vi "File Rename.vi"(10 "name or relative path":string="a.txt", 11 "path":path=path "C:/Users/tilin/Desktop/新文字文件.txt") -> ()   [LabVIEW 2019]
panel:
  out "appended path":path
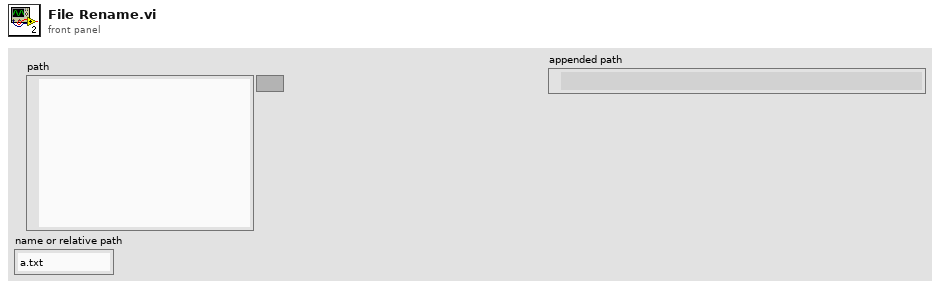
[diagram p1: front panel]
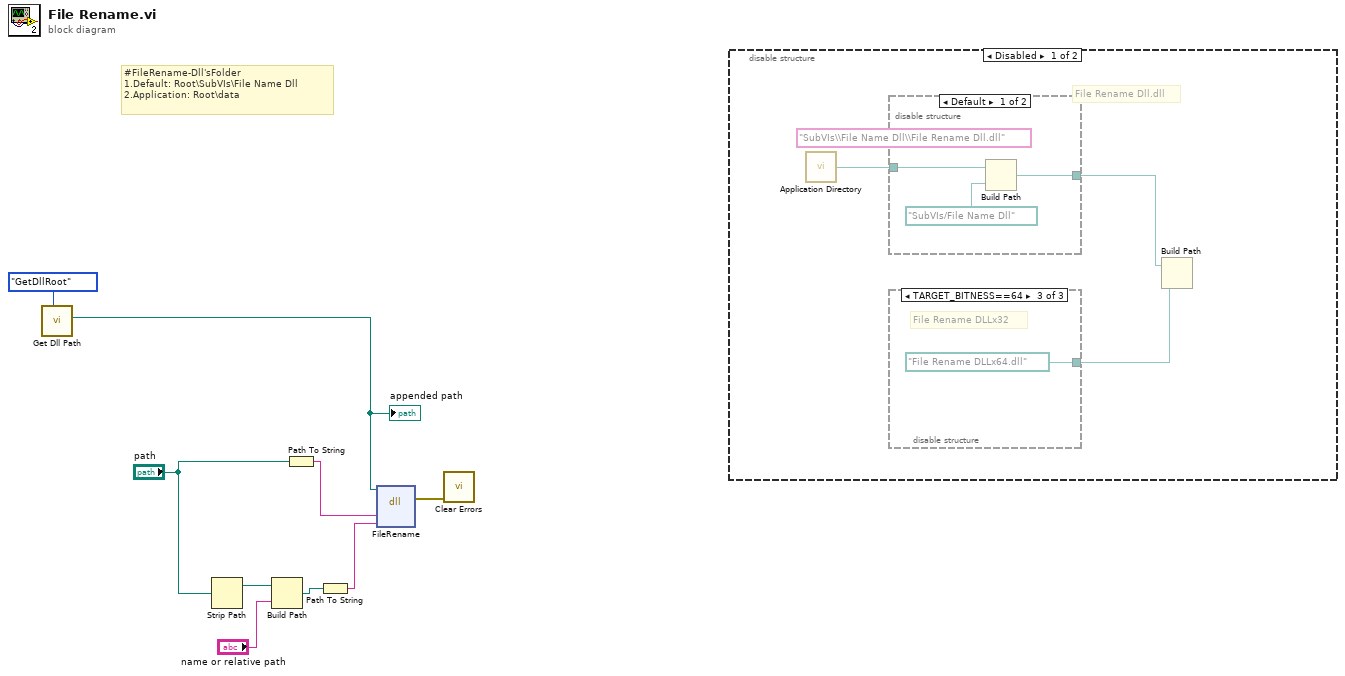
[diagram p0: block diagram]
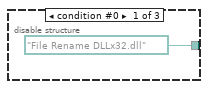
[diagram p2: hidden frame]
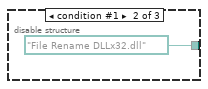
[diagram p3: hidden frame]
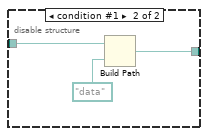
[diagram p4: hidden frame]
diagram:
  # "#FileRename-Dll'sFolder\n1.Default: Root\\SubVIs\\File Name Dll\n2.Application: Root\\data"
  n1 = call "Get Dll Path.vi"("Action"=enum16{"WriteDllRoot", "GetDllRoot"}."GetDllRoot") -> ("Dll Root Path"=w2:path)  [unwired: 10 in]
  "appended path" <- w2
  n2 = Strip Path(path="path") -> (stripped path=w8:path)  [unwired: 1 out]
  n3 = Build Path(base path=w8, name or relative path="name or relative path") -> (appended path=w5:path)
  n4 = Path To String(path="path") -> (string=w6:string)
  n5 = Path To String(path=w5) -> (string=w4:string)
  n6 = dll-call lib="C:/Vision_20160329/SubVIs/File Name Dll/File Rename DLL.dll" fn="FileRename"(path in=w2, "OldName"=w6, "NewName"=w4) -> (error out=w3:errorcluster)  [unwired: 5 in, 1 out]
  n7 = call <vilib>:"Clear Errors.vi"("error in (no error)"=w3) -> ()  [unwired: 5 in, 2 out]
  n8 = disable-structure shown="Disabled" {
    frame Disabled {
      (unwired) "SubVIs\\File Name Dll\\File Rename Dll.dll" ("name or relative path")
      # "File Rename DLLx32"
      # "File Rename Dll.dll"
      n9 = call <vilib>:"Application Directory.vi"() -> ("Application Directory"=w10:path)
      n10 = disable-structure shown="Default" {
        disable-tunnel: w10 -> [w17 w20]
        disable-tunnel: [w16 w19] -> w11
        frame condition #0 (active) {
          n11 = Build Path(base path=w17, name or relative path=path "SubVIs/File Name Dll") -> (appended path=w16:path)
        }
        frame condition #1 {
          n12 = Build Path(base path=w20, name or relative path=path "data") -> (appended path=w19:path)
        }
      }
      n13 = disable-structure shown="TARGET_BITNESS==64" {
        disable-tunnel: [path "File Rename DLLx32.dll" path "File Rename DLLx32.dll" path "File Rename DLLx64.dll"] -> w12
        frame condition #0 {
        }
        frame condition #1 {
        }
        frame condition #2 (active) {
        }
      }
      n14 = Build Path(base path=w11, name or relative path=w12) -> ()  [unwired: 1 out]
    }
    frame Enabled {
    }
  }
